vi "replayer.vi"() -> ()   [LabVIEW 2012]
uses:
  <vilib>/Utility/file.llb/Write To Spreadsheet File (DBL).vi
  G_LCM.vi
panel:
  in  "long format":bool
  out "UDP Comm. Error 2":errorcluster
  out "Receive Buffer Size":u32
  out "recv data":string
  out "Array":string[](array[string])
  out "time":dbl
  out "log time":string
  in  "time-to-live":u16
  out "LCM":T1
  out "Wait for next data recv [sec]":dbl
  out "File Path":path
  in  "배속(0.1~10)":dbl=0.2 min=0.1 max=10.0 step=0.1
  out "t_old":i64
  out "idxtime":i64[](array[numeric])
  in  "Sequence Index Slider":i32(slide) scale=0.0..351997.0
  out "idxsize":i32[](array[numeric])
  in  "Play/Pause":bool
  out "channel":string
  out "header":T2 {"magic" format="%08x"}
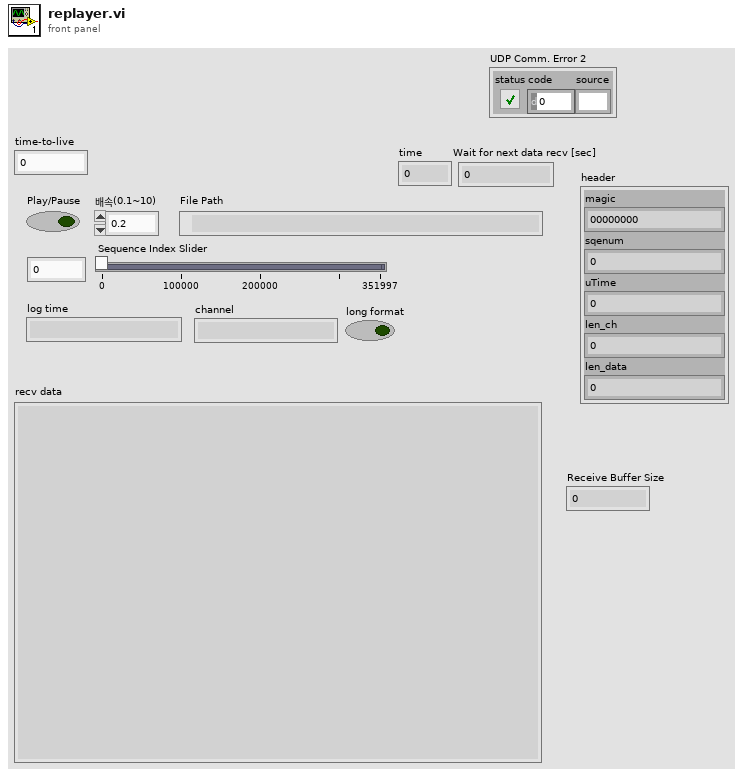
[diagram p1: front panel]
types:
  T1 = cluster{"connection ID":refnum<k16>, "net address":u32, "port":u16}
  T2 = cluster{"magic":i32, "sqenum":i64, "uTime":i64, "len_ch":i32, "len_data":i32}
  T3 = enum8{"Enabled", "Disabled", "Disabled and Grayed Out"}
  T4 = cluster{"hash":i64, "sys time":i64, "time":dbl, "yaw_rate":dbl, "mdps torque":dbl, "mdps str_ang":dbl, "VS_CAN":dbl, "lat_accel":dbl, "mcp":dbl, "accel pedal value":dbl, "tps":dbl, "odometer":dbl, "battery voltage":dbl, "WHL_SPD_RR":dbl, "WHL_SPD_RL":dbl, "WHL_SPD_FR":dbl, "WHL_SPD_FL":dbl}
  T5 = cluster{"hash":dbl, "sys time":dbl, "time":dbl, "yaw_rate":dbl, "mdps torque":dbl, "mdps str_ang":dbl, "VS_CAN":dbl, "lat_accel":dbl, "mcp":dbl, "accel pedal value":dbl, "tps":dbl, "odometer":dbl, "battery voltage":dbl, "WHL_SPD_RR":dbl, "WHL_SPD_RL":dbl, "WHL_SPD_FR":dbl, "WHL_SPD_FL":dbl}
  T6 = cluster{"hash":i64, "sys time":i64, "time":dbl, "x":dbl, "y":dbl, "h":dbl, "numSV":i32, "postype":i32, "lag":i32, "hordev":dbl, "lat":dbl, "lon":dbl, "hgt":dbl, "map_idx":i32}
  T7 = cluster{"hash":dbl, "sys time":dbl, "time":dbl, "x":dbl, "y":dbl, "h":dbl, "numSV":dbl, "postype":dbl, "lag":dbl, "hordev":dbl, "lat":dbl, "lon":dbl, "hgt":dbl, "map_idx":dbl}
  T8 = cluster{"hash":i64, "sys time":i64, "time":dbl, "speed":dbl, "heading":dbl, "lat":dbl, "lon":dbl}
  T9 = cluster{"hash":dbl, "sys time":dbl, "time":dbl, "speed":dbl, "heading":dbl, "lat":dbl, "lon":dbl}
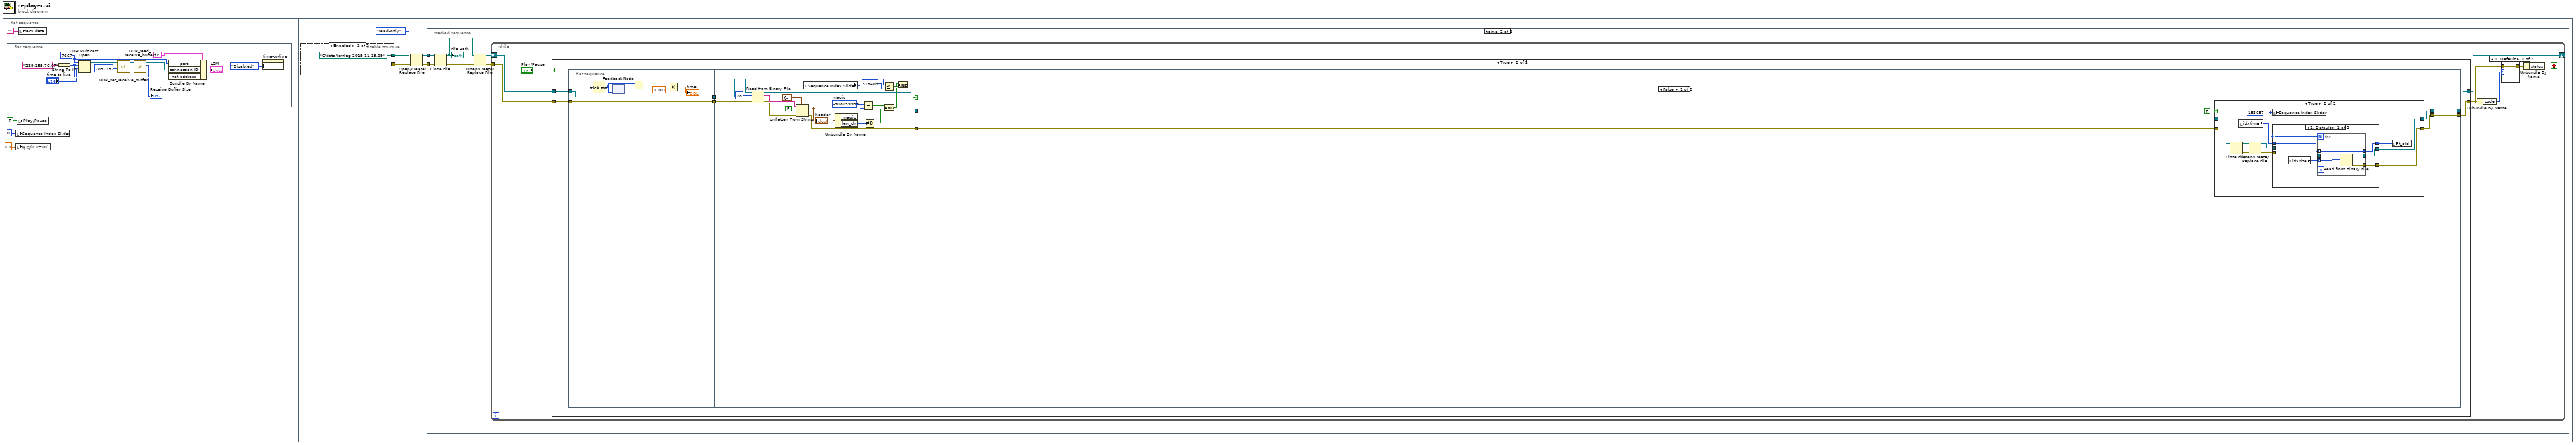
[diagram p0: block diagram]
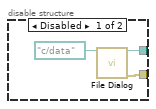
[diagram p2: hidden frame]
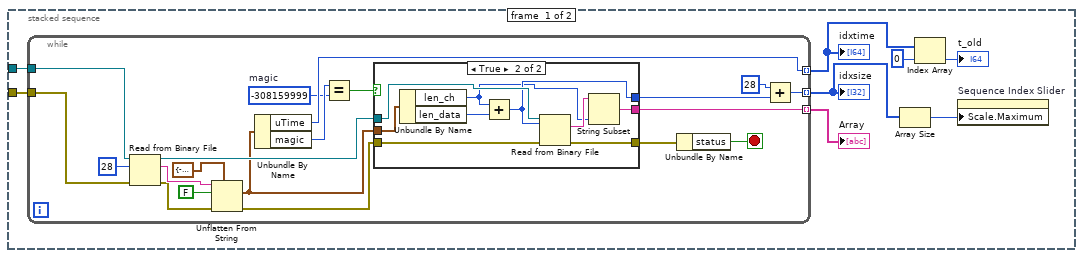
[diagram p3: hidden frame]
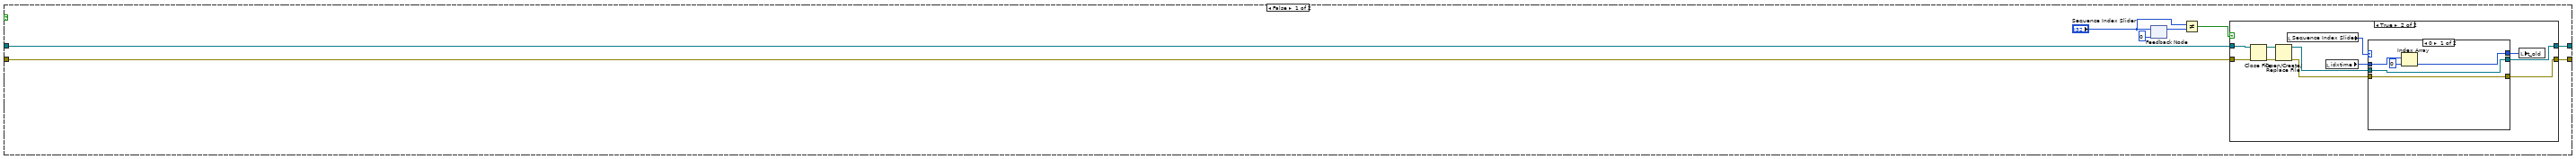
[diagram p6: hidden frame]
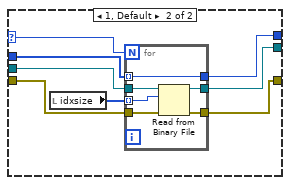
[diagram p8: hidden frame]
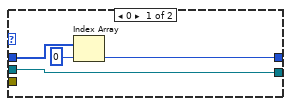
[diagram p10: hidden frame]
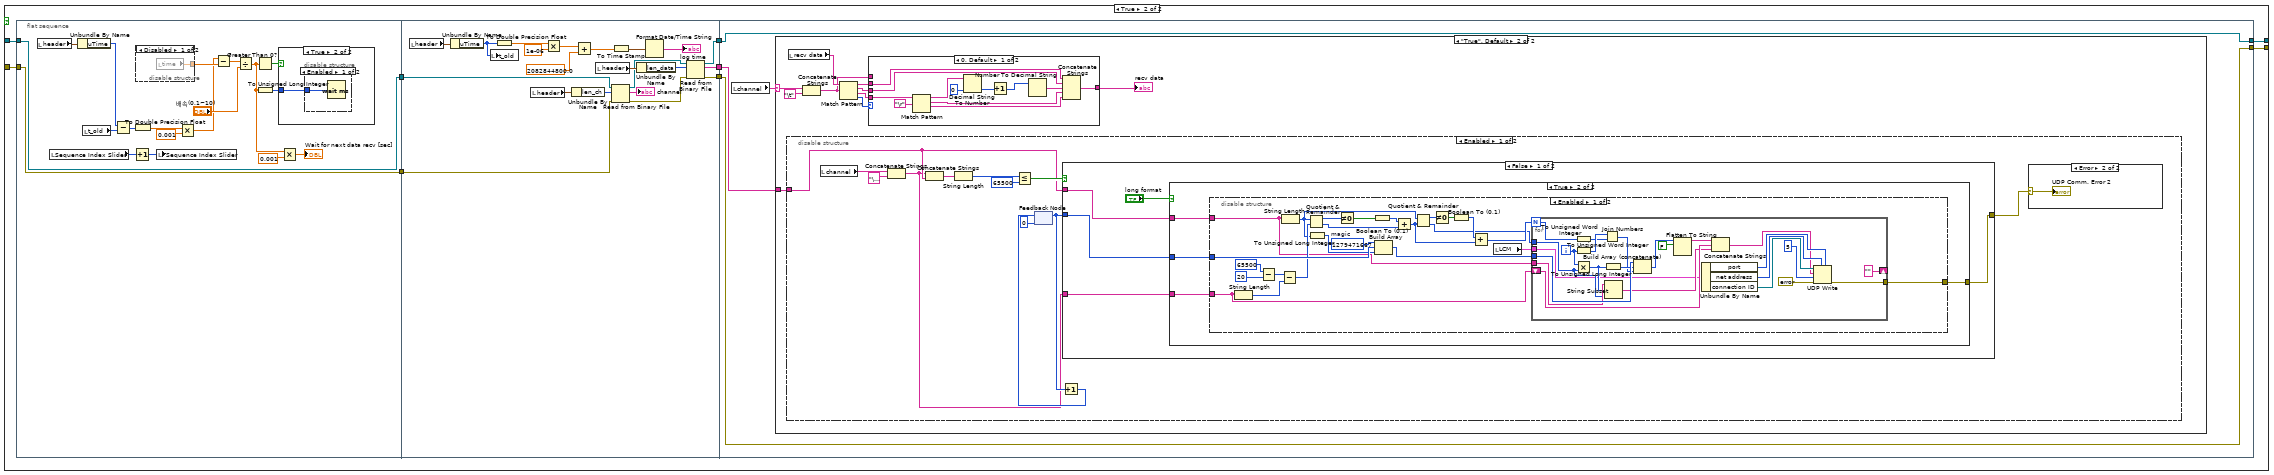
[diagram p11: hidden frame]
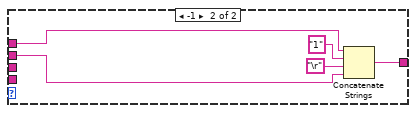
[diagram p16: hidden frame]
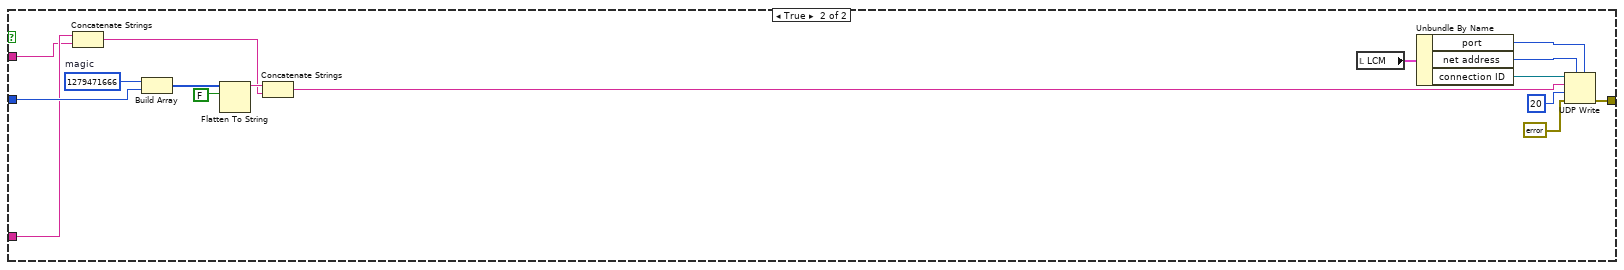
[diagram p19: hidden frame]
diagram:
  n1 = flat-sequence {
    frame #0 {
      n2 = flat-sequence {
        frame #0 {
          w11 = u16 7667 ("port")
          n3 = String To IP(1:"239.255.76.67" ("Multicast Address")) -> (0:w15:u32)
          n4 = UDP Multicast Open(9:"time-to-live", 10:w15, 11:w11) -> (3:w7:refnum<k16>)  [unwired: 2 in, 2 out]
          n5 = call "UDP_set_receive_buffer.vi"("Receive Buffer Size"=u32 2097152, "connection ID"=w7) -> ("error out"=w8:errorcluster, "connection ID out"=w6:refnum<k16>)  [unwired: 7 in]
          n6 = call "UDP_read_receive_buffer.vi"("error in (no error)"=w8, "connection ID"=w6) -> ("Receive Buffer Size"=→"Receive Buffer Size":u32, "connection ID out"=w5:refnum<k16>)  [unwired: 5 in, 1 out]
          n7 = Bundle By Name(cluster=T1 {"connection ID"=refnum, "net address"=0, "port"=7667} ("LCM"), "port"=w11, "connection ID"=w5, "net address"=w15) -> (→"LCM":T1)
        }
        frame #1 {
          n8 = property on="time-to-live" class="DigNum (strict)"("DisabledEnum"=T3."Disabled" ("Disabled")) -> ()  [unwired: 2 in, 2 out]
        }
      }
      n9 = local write "Sequence Index Slider"(0 ("Slide")) -> ()
      n10 = local write "배속(0.1~10)"(1.0 ("배속(0.1~10)")) -> ()
      n11 = local write "Play/Pause"(TRUE ("play")) -> ()
      n12 = local write "recv data"("") -> ()
    }
    frame #1 {
      n13 = disable-structure shown="Enabled" {
        disable-tunnel: [w25 path "C:/data/lcmlog-2015-11-29.09" ("selected path")] -> w19
        disable-tunnel: [w23 _] -> w18
        frame Disabled {
          n14 = call "File Dialog"("start path"=path "c:/data") -> ("selected path"=w25:path, "error out"=w23:errorcluster)  [unwired: 11 in, 2 out]
        }
        frame Enabled {
        }
      }
      n15 = Open/Create/Replace File(file path (use dialog)=w19, error in=w18, access (0:read/write)=enum16{"read/write", "read-only", "write-only"}."read-only") -> (refnum out=w21:refnum<file>, error out=w22:errorcluster)  [unwired: 3 in, 1 out]
      n16 = stacked-sequence {
        tunnel: w21 -> [w34 w70]
        tunnel: w22 -> [w33 w69]
        frame #0 {
          n17 = while {
            tunnel: [w39] -> w32 mode=indexing
            tunnel: w34 -> [w52]
            tunnel: w33 -> [w40]
            tunnel: [w38] -> w30 mode=indexing
            tunnel: [w35] -> w27 mode=indexing
            stop <- w53 stop-if-true
            w36 = -308159999  # magic
            n18 = Read from Binary File(8:w40, 10:28 ("count (1)"), 11:w52) -> (0:w41:errorcluster, 2:w43:string, 3:w51:refnum<file>)  [unwired: 3 in, 1 out]
            n19 = Unflatten From String(type=T2 {"magic"=-308159999, "sqenum"=0, "uTime"=0, "len_ch"=0, "len_data"=0} ("header"), binary string=w43, data includes array or string size? (T)=FALSE, error in (no error)=w41) -> (value=w46:T2, error out=w49:errorcluster)  [unwired: 1 in, 1 out]
            n20 = Unbundle By Name(w46) -> ("uTime"=w38:i64, "magic"=w37:i32)
            n21 = Equal?(x=w37, y=w36) -> (x = y?=w50:bool)
            n22 = case shown="True" w50 {
              tunnel: w51 -> [_ w64]
              tunnel: [w55 w62] -> w54
              tunnel: w49 -> [w55 w63]
              tunnel: [_ w61] -> w48
              tunnel: w46 -> [_ w59]
              tunnel: [_ w56] -> w35
              frame False {
              }
              frame True {
                n23 = Unbundle By Name(w59) -> ("len_ch"=w57:i32, "len_data"=w60:i32)
                n24 = Add(x=w57, y=w60) -> (x+y=w61:i32)
                n25 = Read from Binary File(8:w63, 10:w61, 11:w64) -> (0:w62:errorcluster, 2:w58:string)  [unwired: 3 in, 2 out]
                n26 = String Subset(string=w58, length (rest)=w57) -> (substring=w56:string)  [unwired: 1 in]
              }
            }
            n27 = Unbundle By Name(w54) -> ("status"=w53:bool)
            n28 = Add(x=28 ("count (1)"), y=w48) -> (x+y=w39:i32)
          }
          "idxsize" <- w32
          "idxtime" <- w30
          "Array" <- w27
          n29 = Array Size(array=w32) -> (size(s)=w31:i32)
          n30 = Index Array(array=w30, index=0) -> (element=→"t_old":i64)
          n31 = property on="Sequence Index Slider" class="Slide (strict)"("Scale.Maximum"=w31) -> ()  [unwired: 2 in, 2 out]
        }
        frame #1 {
          n32 = Close File(refnum=w70, error in=w69) -> (path=w67:path, error out=w68:errorcluster)
          "File Path" <- w67
          n33 = Open/Create/Replace File(file path (use dialog)=w67, error in=w68) -> (refnum out=w66:refnum<file>, error out=w65:errorcluster)  [unwired: 4 in, 1 out]
          n34 = while {
            tunnel: w65 -> [w75]
            shift-right: [w74] -> _
            shift-left: w66 -> [w78]
            stop <- w77 stop-if-true
            n35 = case shown="True" "Play/Pause" {
              tunnel: w78 -> [w85 w125]
              tunnel: [w82 w124] -> w71
              tunnel: w75 -> [w84 w123]
              tunnel: [w83 w122] -> w74
              frame False {
                n36 = feedback-in #1("Sequence Index Slider") -> ()
                n37 = feedback #1(0 ("Slide")) -> (w80:i32)
                n38 = Not Equal?(x="Sequence Index Slider", y=w80) -> (x != y?=w86:bool)
                n39 = case shown="True" w86 {
                  tunnel: w85 -> [w89 w98]
                  tunnel: w84 -> [w88 w97]
                  tunnel: [w89 w94] -> w83
                  tunnel: [w88 w93] -> w82
                  frame False {
                  }
                  frame True {
                    n40 = Close File(refnum=w98, error in=w97) -> (path=w99:path, error out=w100:errorcluster)
                    n41 = Open/Create/Replace File(file path (use dialog)=w99, error in=w100) -> (refnum out=w96:refnum<file>, error out=w95:errorcluster)  [unwired: 4 in, 1 out]
                    n42 = local read "Sequence Index Slider"() -> (w90:i32)
                    n43 = local read "idxtime"() -> (w91:i64[])
                    n44 = case shown="0" w90 {
                      selector: w90 -> [_ w106]
                      tunnel: w96 -> [w103 w113]
                      tunnel: w95 -> [w102 w112]
                      tunnel: [w103 w110] -> w94
                      tunnel: [w102 w109] -> w93
                      tunnel: [w104 w108] -> w92
                      tunnel: w91 -> [w105 w107]
                      frame 0 {
                        n45 = Index Array(array=w105, index=0) -> (element=w104:i64)
                      }
                      frame 1, Default {
                        n46 = local read "idxsize"() -> (w111:i32[])
                        n47 = for {
                          N: w106 -> [_]
                          tunnel: w113 -> [w119]
                          tunnel: w112 -> [w118]
                          tunnel: w111 -> [w117] mode=indexing
                          tunnel: [w116] -> w110
                          tunnel: [w115] -> w109
                          tunnel: [w114] -> w108
                          tunnel: w107 -> [w114] mode=indexing
                          n48 = Read from Binary File(8:w118, 10:w117, 11:w119) -> (0:w115:errorcluster, 3:w116:refnum<file>)  [unwired: 3 in, 2 out]
                        }
                      }
                    }
                    n49 = local write "t_old"(w92) -> ()
                  }
                }
              }
              frame True {
                n50 = flat-sequence {
                  tunnel: w123 -> [w131]
                  tunnel: w125 -> [w132]
                  tunnel: [w132] -> w121
                  tunnel: [w131] -> w120
                  tunnel: [w153] -> w124
                  tunnel: [w151] -> w122
                  tunnel: w121 -> [w154]
                  tunnel: w120 -> [w152]
                  frame #0 {
                    n51 = Tick Count (ms)() -> (millisecond timer value=w129:u32)
                    n52 = feedback-in #2(w129) -> ()
                    n53 = feedback #2(w129) -> (w130:u32)
                    n54 = Subtract(x=w129, y=w130) -> (x-y=w128:u32)
                    n55 = Multiply(x=w128, y=0.001) -> (x*y=→"time":dbl)
                  }
                  frame #1 {
                    w142 = -308159999  # magic
                    n56 = Read from Binary File(8:w152, 10:28 ("count (1)"), 11:w154) -> (0:w144:errorcluster, 2:w146:string, 3:w150:refnum<file>)  [unwired: 3 in, 1 out]
                    n57 = Unflatten From String(type=T2 {"magic"=-308159999, "sqenum"=0, "uTime"=0, "len_ch"=0, "len_data"=0} ("header"), binary string=w146, data includes array or string size? (T)=FALSE, error in (no error)=w144) -> (value=w143:T2, error out=w149:errorcluster)  [unwired: 1 in, 1 out]
                    "header" <- w143
                    n58 = local read "Sequence Index Slider"() -> (w137:i32)
                    n59 = Unbundle By Name(w143) -> ("magic"=w141:i32, "len_ch"=w140:i32)
                    n60 = Equal?(x=w142, y=w141) -> (x = y?=w138:bool)
                    n61 = Not Equal To 0?(x=w140) -> (x != 0?=w139:bool)
                    n62 = Less Or Equal?(x=w137, y=318403) -> (x <= y?=w135:bool)
                    n63 = And(x=w138, y=w139) -> (x .and. y?=w134:bool)
                    n64 = And(x=w134, y=w135) -> (x .and. y?=w133:bool)
                    n65 = case shown="False" w133 {
                      tunnel: w150 -> [w159 w196]
                      tunnel: [w156 w192] -> w153
                      tunnel: w149 -> [w158 w193]
                      tunnel: [w157 w191] -> w151
                      frame False {
                        n66 = case shown="True" TRUE {
                          tunnel: w159 -> [w161 w169]
                          tunnel: w158 -> [w160 _]
                          tunnel: [w161 w166] -> w157
                          tunnel: [w160 w165] -> w156
                          frame False {
                          }
                          frame True {
                            w162 = 183687 ("Sequence Index Slider")
                            n67 = Close File(refnum=w169) -> (path=w170:path, error out=w171:errorcluster)  [unwired: 1 in]
                            n68 = local read "idxtime"() -> (w163:i64[])
                            n69 = Open/Create/Replace File(file path (use dialog)=w170, error in=w171) -> (refnum out=w168:refnum<file>, error out=w167:errorcluster)  [unwired: 4 in, 1 out]
                            n70 = local write "Sequence Index Slider"(w162) -> ()
                            n71 = case shown="1, Default" w162 {
                              selector: w162 -> [_ w176]
                              tunnel: w168 -> [w173 w182]
                              tunnel: w167 -> [_ _]
                              tunnel: [w173 w180] -> w166
                              tunnel: [_ w179] -> w165
                              tunnel: [w174 w178] -> w164
                              tunnel: w163 -> [w175 w177]
                              frame 0 {
                                n72 = Index Array(array=w175, index=0) -> (element=w174:i64)
                              }
                              frame 1, Default {
                                n73 = local read "idxsize"() -> (w181:i32[])
                                n74 = for {
                                N: w176 -> [_]
                                tunnel: w182 -> [w187]
                                tunnel: w181 -> [w186] mode=indexing
                                tunnel: [w185] -> w180
                                tunnel: [w184] -> w179
                                tunnel: [w183] -> w178
                                tunnel: w177 -> [w183] mode=indexing
                                n75 = Read from Binary File(10:w186, 11:w187) -> (0:w184:errorcluster, 3:w185:refnum<file>)  [unwired: 4 in, 2 out]
                                }
                              }
                            }
                            n76 = local write "t_old"(w164) -> ()
                          }
                        }
                      }
                      frame True {
                        n77 = flat-sequence {
                          tunnel: [w215] -> w195
                          tunnel: [w209] -> w194
                          tunnel: w196 -> [w215]
                          tunnel: w193 -> [w209]
                          tunnel: w195 -> [w239]
                          tunnel: w194 -> [w227]
                          tunnel: [w221] -> w190
                          tunnel: [w226] -> w189
                          tunnel: [w222] -> w188
                          tunnel: [w242] -> w191
                          tunnel: [w243] -> w192
                          tunnel: w190 -> [w243]
                          tunnel: w189 -> [w242]
                          tunnel: w188 -> [w241]
                          frame #0 {
                            n78 = local read "header"() -> (w213:T2)
                            n79 = local read "Sequence Index Slider"() -> (w203:i32)
                            n80 = Unbundle By Name(w213) -> ("uTime"=w214:i64)
                            n81 = local read "t_old"() -> (w208:i64)
                            n82 = Subtract(x=w214, y=w208) -> (x-y=w212:i64)
                            n83 = Increment(x=w203) -> (x+1=w204:i32)
                            n84 = To Double Precision Float(number=w212) -> (double precision float=w210:dbl)
                            n85 = disable-structure shown="Disabled" {
                              disable-tunnel: [w216 _] -> w199
                              frame Disabled {
                                n86 = local read "time"() -> (w216:dbl)
                              }
                              frame Enabled {
                              }
                            }
                            n87 = local write "Sequence Index Slider"(w204) -> ()
                            n88 = Multiply(x=w210, y=0.001) -> (x*y=w198:dbl)
                            n89 = Subtract(x=w198, y=w199) -> (x-y=w197:dbl)
                            n90 = Divide(x=w197, y="배속(0.1~10)") -> (x/y=w201:dbl)
                            n91 = Greater Than 0?(x=w201) -> (x > 0?=w200:bool)
                            n92 = To Unsigned Long Integer(number=w201) -> (unsigned 32bit integer=w202:u32)
                            n93 = case shown="True" w200 {
                              tunnel: w202 -> [_ w217]
                              frame False {
                              }
                              frame True {
                                n94 = disable-structure shown="Enabled" {
                                disable-tunnel: w217 -> [w218 _]
                                frame Enabled {
                                n95 = Wait (ms)(milliseconds to wait=w218) -> ()  [unwired: 1 out]
                                }
                                frame Disabled {
                                }
                                }
                              }
                            }
                            n96 = Multiply(x=w201, y=0.001) -> (x*y=→"Wait for next data recv [sec]":dbl)
                          }
                          frame #1 {
                            n97 = local read "header"() -> (w230:T2)
                            n98 = Unbundle By Name(w230) -> ("uTime"=w225:i64)
                            n99 = local write "t_old"(w225) -> ()
                            n100 = To Double Precision Float(number=w225) -> (double precision float=w234:dbl)
                            n101 = local read "header"() -> (w238:T2)
                            n102 = Multiply(x=w234, y=1e-06) -> (x*y=w232:dbl)
                            n103 = Unbundle By Name(w238) -> ("len_ch"=w237:i32)
                            n104 = Add(x=w232, y=2082844800.0 ("UTC+9h from 1970-01-01")) -> (x+y=w235:dbl)
                            n105 = local read "header"() -> (w229:T2)
                            n106 = Read from Binary File(8:w227, 10:w237, 11:w239) -> (0:w220:errorcluster, 2:→"channel":string, 3:w228:refnum<file>)  [unwired: 3 in, 1 out]
                            n107 = To Time Stamp(1:w235) -> (0:w224:timestamp)
                            n108 = Unbundle By Name(w229) -> ("len_data"=w219:i32)
                            n109 = Format Date/Time String(seconds (now)=w224) -> (date/time string=→"log time":string)  [unwired: 2 in]
                            n110 = Read from Binary File(8:w220, 10:w219, 11:w228) -> (0:w221:errorcluster, 2:w222:string, 3:w226:refnum<file>)  [unwired: 3 in, 1 out]
                          }
                          frame #2 {
                            n111 = local read "channel"() -> (w240:string)
                            n112 = case shown="\"True\", Default" w240 {
                              selector: w240 -> [_ w245]
                              tunnel: w241 -> [_ w244]
                              frame "" {
                              }
                              frame "True", Default {
                                n113 = disable-structure shown="Enabled" {
                                disable-tunnel: w244 -> [w272 w358]
                                frame Enabled {
                                n114 = local read "channel"() -> (w278:string)
                                n115 = Concatenate Strings(w278, "\u0000" ("string")) -> (w271:string)
                                n116 = Concatenate Strings(w271, w272) -> (w273:string)
                                n117 = String Length(string=w273) -> (length=w276:i32)
                                n118 = Less Or Equal?(x=w276, y=65500 ("length (rest)")) -> (x <= y?=w274:bool)
                                n119 = feedback #3(u32 0) -> (w281:u32)
                                n120 = Increment(x=w281) -> (x+1=w282:u32)
                                n121 = feedback-in #3(w282) -> ()
                                n122 = case shown="False" w274 {
                                tunnel: w281 -> [w287 w354]
                                tunnel: [w284 w345] -> w279
                                tunnel: w272 -> [w285 w341]
                                tunnel: w271 -> [w286 w342]
                                frame False {
                                n123 = case shown="True" "long format" {
                                tunnel: w287 -> [_ w291]
                                tunnel: w286 -> [_ w290]
                                tunnel: w285 -> [_ w289]
                                tunnel: [_ w288] -> w284
                                frame False {
                                }
                                frame True {
                                n124 = disable-structure shown="Enabled" {
                                disable-tunnel: w291 -> [w314 _]
                                disable-tunnel: w290 -> [w304 _]
                                disable-tunnel: w289 -> [w303 _]
                                disable-tunnel: [w293 _] -> w288
                                frame Enabled {
                                w315 = u32 1279471667  # magic
                                n125 = String Length(string=w304) -> (length=w305:i32)
                                n126 = Subtract(x=65500 ("length (rest)"), y=20) -> (x-y=w308:i32)
                                n127 = Subtract(x=w308, y=w305) -> (x-y=w307:i32)
                                n128 = String Length(string=w303) -> (length=w302:i32)
                                n129 = Quotient & Remainder(x=w302, y=w307) -> (x-y*floor(x/y)=w298:i32, floor(x/y)=w296:i32)
                                n130 = To Unsigned Long Integer(number=w302) -> (unsigned 32bit integer=w310:u32)
                                n131 = Not Equal To 0?(x=w298) -> (x != 0?=w311:bool)
                                n132 = Boolean To (0,1)(Boolean=w311) -> (0, 1=w297:i16)
                                n133 = Build Array(w315, w314, w310) -> (w306:u32[])
                                n134 = Add(x=w297, y=w296) -> (x+y=w300:i32)
                                n135 = Quotient & Remainder(x=w302, y=w300) -> (x-y*floor(x/y)=w294:i32, floor(x/y)=w295:i32)
                                n136 = Not Equal To 0?(x=w294) -> (x != 0?=w309:bool)
                                n137 = Boolean To (0,1)(Boolean=w309) -> (0, 1=w301:i16)
                                n138 = Add(x=w301, y=w300) -> (x+y=w299:i32)
                                n139 = local read "LCM"() -> (w292:T1)
                                n140 = for {
                                N: w299 -> [w337]
                                tunnel: w295 -> [w325]
                                tunnel: w306 -> [w339]
                                shift-right: [""] -> _
                                shift-left: w304 -> [w328]
                                tunnel: w303 -> [w332]
                                tunnel: [w317] -> w293
                                tunnel: w292 -> [w316]
                                i -> [w324]
                                n141 = To Unsigned Word Integer(number=w337) -> (unsigned 16bit integer=w335:u16)
                                n142 = To Unsigned Word Integer(number=w324) -> (unsigned 16bit integer=w336:u16)
                                n143 = Multiply(x=w324, y=w325) -> (x*y=w326:i32)
                                n144 = Join Numbers(hi=w336, lo=w335) -> ((hi.lo)=w334:u32)
                                n145 = To Unsigned Long Integer(number=w326) -> (unsigned 32bit integer=w338:u32)
                                n146 = String Subset(string=w332, offset (0)=w326, length (rest)=w325) -> (substring=w327:string)
                                n147 = Build Array (concatenate)(w339, w338, w334) -> (w330:u32[])
                                n148 = Flatten To String(anything=w330, prepend array or string size? (T)=FALSE) -> (data string=w329:string)  [unwired: 2 in, 2 out]
                                n149 = Unbundle By Name(w316) -> ("port"=w321:u16, "net address"=w320:u32, "connection ID"=w319:refnum<k16>)
                                n150 = Concatenate Strings(w329, w328, w327) -> (w318:string)
                                n151 = UDP Write(address=w320, port or service name=w321, connection ID=w319, data in=w318, 8:errorcluster {"status"=FALSE, "code"=0, "source"=""} ("error in (no error)"), 9:5 ("timeout ms (25000)")) -> (error out=w317:errorcluster)  [unwired: 1 out]
                                }
                                }
                                frame Disabled {
                                }
                                }
                                }
                                }
                                }
                                frame True {
                                w351 = u32 1279471666  # magic
                                n152 = Concatenate Strings(w342, w341) -> (w340:string)
                                n153 = Build Array(w351, w354) -> (w352:u32[])
                                n154 = Flatten To String(anything=w352, prepend array or string size? (T)=FALSE) -> (data string=w344:string)  [unwired: 2 in, 2 out]
                                n155 = Concatenate Strings(w344, w340) -> (w343:string)
                                n156 = local read "LCM"() -> (w349:T1)
                                n157 = Unbundle By Name(w349) -> ("port"=w348:u16, "net address"=w347:u32, "connection ID"=w346:refnum<k16>)
                                n158 = UDP Write(address=w347, port or service name=w348, connection ID=w346, data in=w343, 8:errorcluster {"status"=FALSE, "code"=0, "source"=""} ("error in (no error)"), 9:20 ("timeout ms (25000)")) -> (error out=w345:errorcluster)  [unwired: 1 out]
                                }
                                }
                                n159 = case shown="Error" w279 {
                                selector: w279 -> [_ w356]
                                frame No Error {
                                }
                                frame Error {
                                "UDP Comm. Error 2" <- w356
                                }
                                }
                                }
                                frame Disabled {
                                n160 = local read "channel"() -> (w357:string)
                                n161 = case shown="\"RMC_2\"" w357 {
                                tunnel: w358 -> [_ w361 w370 w379 w388 w397]
                                tunnel: [_ w359 w368 w377 w386 w395] -> _
                                frame "False", Default {
                                }
                                frame "CAN_T" {
                                n162 = global read "G_LCM.vi" "CAN_T"() -> (w360:T4)
                                n163 = Unflatten From String(type=w360, binary string=w361, data includes array or string size? (T)=FALSE) -> (value=w366:T4, error out=w359:errorcluster)  [unwired: 2 in, 1 out]
                                n164 = To Double Precision Float(number=w366) -> (double precision float=w365:T5)
                                n165 = Cluster To Array(cluster=w365) -> (array=w364:dbl[])
                                n166 = call-poly <vilib>:"Write To Spreadsheet File.vi"("format (%.3f)"="%.6f", "1D data"=w364, "file path (dialog if empty)"=path "c:/data/can.cvs") -> ()  [unwired: 5 in, 1 out]
                                }
                                frame "GGA_1" {
                                n167 = global read "G_LCM.vi" "GGA_1"() -> (w369:T6)
                                n168 = Unflatten From String(type=w369, binary string=w370, data includes array or string size? (T)=FALSE) -> (value=w375:T6, error out=w368:errorcluster)  [unwired: 2 in, 1 out]
                                n169 = To Double Precision Float(number=w375) -> (double precision float=w374:T7)
                                n170 = Cluster To Array(cluster=w374) -> (array=w373:dbl[])
                                n171 = call-poly <vilib>:"Write To Spreadsheet File.vi"("format (%.3f)"="%.6f", "1D data"=w373, "file path (dialog if empty)"=path "c:/data/gga1.cvs") -> ()  [unwired: 5 in, 1 out]
                                }
                                frame "GGA_2" {
                                n172 = global read "G_LCM.vi" "GGA_2"() -> (w378:T6)
                                n173 = Unflatten From String(type=w378, binary string=w379, data includes array or string size? (T)=FALSE) -> (value=w384:T6, error out=w377:errorcluster)  [unwired: 2 in, 1 out]
                                n174 = To Double Precision Float(number=w384) -> (double precision float=w383:T7)
                                n175 = Cluster To Array(cluster=w383) -> (array=w382:dbl[])
                                n176 = call-poly <vilib>:"Write To Spreadsheet File.vi"("format (%.3f)"="%.6f", "1D data"=w382, "file path (dialog if empty)"=path "c:/data/gga2.cvs") -> ()  [unwired: 5 in, 1 out]
                                }
                                frame "RMC_1" {
                                n177 = global read "G_LCM.vi" "RMC_1"() -> (w387:T8)
                                n178 = Unflatten From String(type=w387, binary string=w388, data includes array or string size? (T)=FALSE) -> (value=w393:T8, error out=w386:errorcluster)  [unwired: 2 in, 1 out]
                                n179 = To Double Precision Float(number=w393) -> (double precision float=w392:T9)
                                n180 = Cluster To Array(cluster=w392) -> (array=w391:dbl[])
                                n181 = call-poly <vilib>:"Write To Spreadsheet File.vi"("format (%.3f)"="%.6f", "1D data"=w391, "file path (dialog if empty)"=path "c:/data/rmc1.cvs") -> ()  [unwired: 5 in, 1 out]
                                }
                                frame "RMC_2" {
                                n182 = global read "G_LCM.vi" "RMC_2"() -> (w396:T8)
                                n183 = Unflatten From String(type=w396, binary string=w397, data includes array or string size? (T)=FALSE) -> (value=w402:T8, error out=w395:errorcluster)  [unwired: 2 in, 1 out]
                                n184 = To Double Precision Float(number=w402) -> (double precision float=w401:T9)
                                n185 = Cluster To Array(cluster=w401) -> (array=w400:dbl[])
                                n186 = call-poly <vilib>:"Write To Spreadsheet File.vi"("format (%.3f)"="%.6f", "1D data"=w400, "file path (dialog if empty)"=path "c:/data/rmc2.cvs") -> ()  [unwired: 5 in, 1 out]
                                }
                                }
                                }
                                }
                                n187 = local read "recv data"() -> (w251:string)
                                n188 = Concatenate Strings(w245, "\t") -> (w247:string)
                                n189 = Match Pattern(string=w251, regular expression=w247) -> (before substring=w250:string, match substring=w249:string, after substring=w248:string, offset past match=w253:i32)  [unwired: 1 in]
                                n190 = case shown="0, Default" w253 {
                                tunnel: [w261 w270] -> w252
                                tunnel: w250 -> [w256 w266]
                                tunnel: w249 -> [w255 _]
                                tunnel: w248 -> [w254 _]
                                tunnel: w247 -> [_ w267]
                                frame 0, Default {
                                n191 = Match Pattern(string=w254, regular expression="\r") -> (before substring=w265:string, match substring=w263:string, after substring=w264:string)  [unwired: 1 in, 1 out]
                                n192 = Decimal String To Number(string=w265, default (0L)=u64 0 ("default (0 I32)")) -> (number=w258:u64)  [unwired: 1 in, 1 out]
                                n193 = Increment(x=w258) -> (x+1=w260:u64)
                                n194 = Number To Decimal String(number=w260) -> (decimal integer string=w259:string)  [unwired: 1 in]
                                n195 = Concatenate Strings(w256, w255, w259, w263, w264) -> (w261:string)
                                }
                                frame -1 {
                                n196 = Concatenate Strings(w267, "1", "\r", w266) -> (w270:string)
                                }
                                }
                                "recv data" <- w252
                              }
                            }
                          }
                        }
                      }
                    }
                  }
                }
              }
            }
            n197 = Unbundle By Name(w71) -> ("code"=w73:i32)
            n198 = case shown="0, Default" w73 {
              tunnel: [w79 _] -> w72
              tunnel: w71 -> [w79 _]
              frame 0, Default {
              }
              frame 4 {
              }
            }
            n199 = Unbundle By Name(w72) -> ("status"=w77:bool)
          }
        }
      }
    }
  }
